vi "Turret_Execute.vi"() -> ()   [LabVIEW 2019]
uses:
  Turret_States.ctl
  Utility VIs/Basic_Motor_Modes.ctl
  Globals/Turret_Globals.vi
  Globals/Sensor_Values.vi
panel:
  in  "Disable Edge Safeties?":bool
  out "Waveform Chart":cluster{"Goal Wheel Position":dbl, dbl}(graph)
  in  "Kp_Degrees":dbl=0.07
  in  "Kd Aim":dbl=0.001
  in  "Ki Aim":dbl=1e-05
  out "Turret_Spin_Speed":dbl
  in  "Kp Aim":dbl=0.06
  # "e"
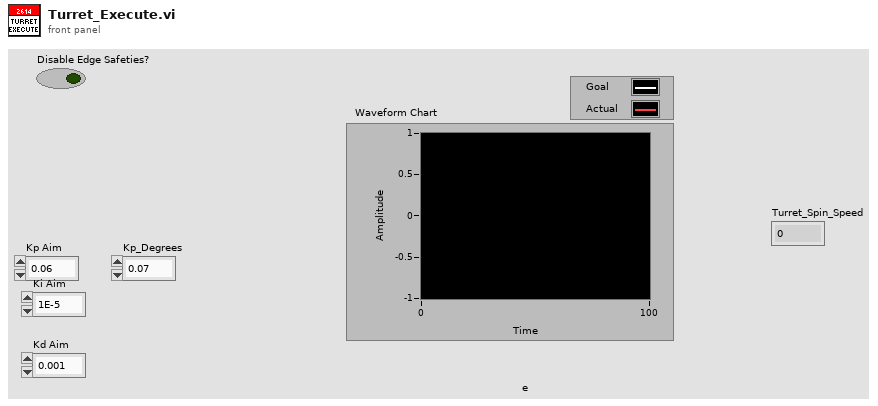
[diagram p1: front panel]
types:
  T1 = typedef "Turret_States.ctl" = enum16{"Manual_Percent_Voltage", "Manual_Speed_Control", "Auto-Target", "Command_TurnToPosition", "Command_Auto_Target", "GoToZero"}
  T2 = typedef "Basic_Motor_Modes.ctl" = enum16{"Percent_Voltage", "Speed_Control", "Position_Control", "Current"}
  T3 = typedef "Turret_Cluster.ctl" = cluster{"Auto-Target?":bool, "Control_State":T1, "Turret_Spin_Speed":dbl, "Turret_Spin_Speed_Control?":bool, "Step":dbl, "Auto_Notifier":refnum<notifier>, "GoToZero?":bool, "Parameters":dbl[]}
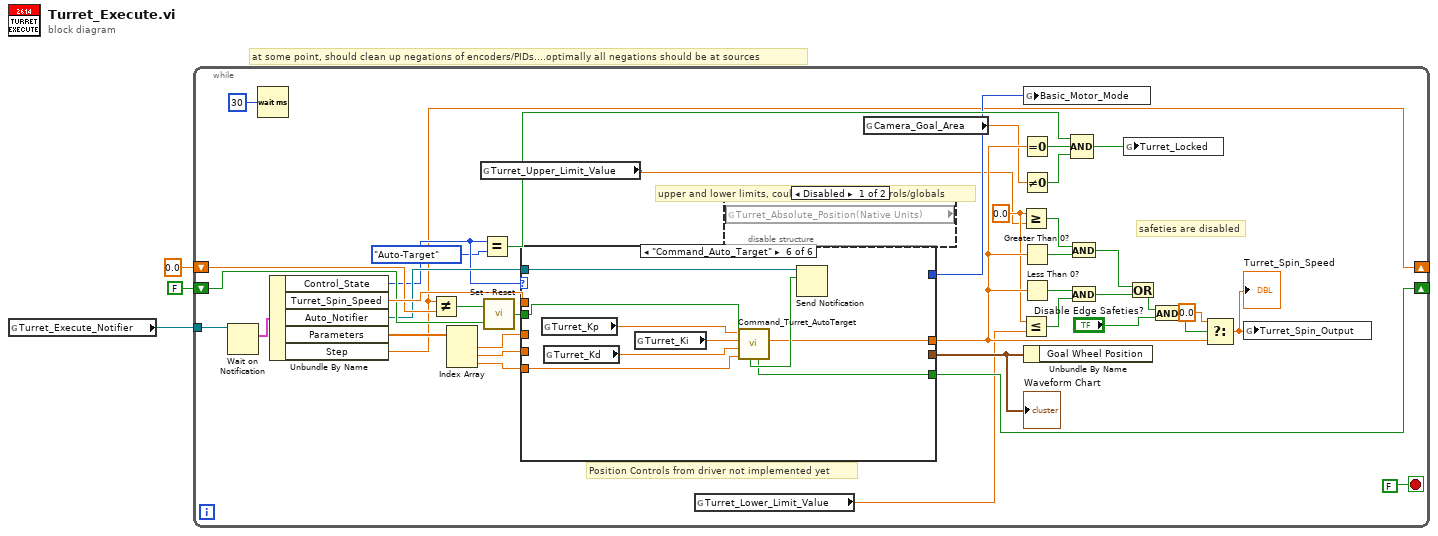
[diagram p0: block diagram]
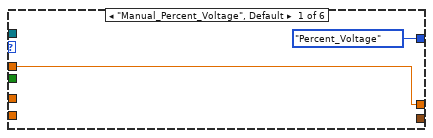
[diagram p3: hidden frame]
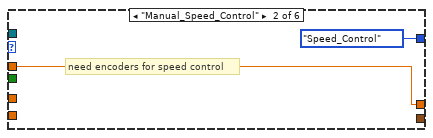
[diagram p4: hidden frame]
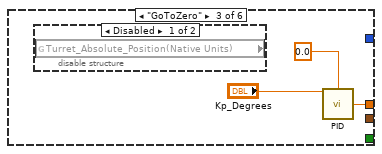
[diagram p5: hidden frame]
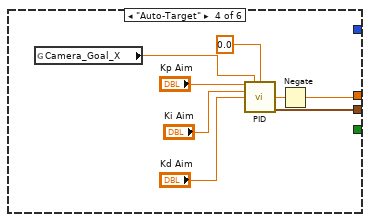
[diagram p7: hidden frame]
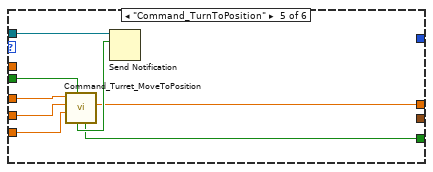
[diagram p8: hidden frame]
diagram:
  # "at some point, should clean up negations of encoders/PIDs....optimally all negations should be at sources"
  n1 = global read "Turret_Globals.vi" "Turret_Execute_Notifier"() -> (w3:refnum<notifier>)
  n2 = while {
    tunnel: w3 -> [w42]
    shift-right: [w6] -> _
    shift-left: 0.0 ("Step") -> [w31]
    shift-right: [w25] -> _
    shift-left: FALSE ("Output") -> [w29]
    stop <- FALSE stop-if-true
    w10 = 0.0 ("x")
    # "safeties are disabled"
    # "Position Controls from driver not implemented yet"
    # "upper and lower limits, could be made into controls/globals"
    n3 = Wait on Notification(notifier=w42) -> (notification=w41:T3)  [unwired: 3 in, 3 out]
    n4 = Wait (ms)(milliseconds to wait=u32 30) -> ()  [unwired: 1 out]
    n5 = Unbundle By Name(w41) -> ("Control_State"=w24:T1, "Turret_Spin_Speed"=w40:dbl, "Auto_Notifier"=w26:refnum<notifier>, "Parameters"=w28:dbl[], "Step"=w6:dbl)
    n6 = Not Equal?(x=w6, y=w31) -> (x != y?=w30:bool)
    n7 = Index Array(array=w28) -> (element #1=w9:dbl, element #2=w8:dbl, element #3=w7:dbl)  [unwired: 3 in]
    n8 = global read "Sensor_Values.vi" "Turret_Upper_Limit_Value"() -> (w5:dbl)
    n9 = Equal?(x=w24, y=Turret_States."Auto-Target") -> (x = y?=w20:bool)
    n10 = call "Set - Reset.vi"("Reset"=w29, "Set"=w30) -> ("Output"=w27:bool)
    n11 = case shown="\"Command_Auto_Target\"" w24 {
      tunnel: w40 -> [w45 w47 _ _ _ _]
      tunnel: [w45 w47 w48 w51 w59 w70] -> w22
      tunnel: w9 -> [_ _ _ _ w66 _]
      tunnel: w8 -> [_ _ _ _ w65 _]
      tunnel: w7 -> [_ _ _ _ w64 w75]
      tunnel: w27 -> [_ _ _ _ w63 w74]
      tunnel: w26 -> [_ _ _ _ w62 w73]
      tunnel: [_ _ _ _ w60 w71] -> w25
      tunnel: [_ _ _ w53 _ _] -> w16
      tunnel: [Basic_Motor_Modes."Percent_Voltage" ("Motor_Mode") Basic_Motor_Modes."Speed_Control" ("Motor_Mode") _ _ _ _] -> w14
      frame "Manual_Percent_Voltage", Default {
      }
      frame "Manual_Speed_Control" {
        # "need encoders for speed control"
      }
      frame "GoToZero" {
        n12 = disable-structure shown="Disabled" {
          frame Disabled {
            n13 = global read "Sensor_Values.vi" "Turret_Absolute_Position(Native Units)"() -> ()  [unwired: 1 out]
          }
          frame Enabled {
          }
        }
        n14 = call "PID.vi"("Kp"="Kp_Degrees", "Goal"=0.0) -> ("Command"=w48:dbl)  [unwired: 11 in, 2 out]
      }
      frame "Auto-Target" {
        n15 = global read "Sensor_Values.vi" "Camera_Goal_X"() -> (w56:dbl)
        n16 = call "PID.vi"("Kp"="Kp Aim", "Process Variable"=w56, "Goal"=0.0, "Ki"="Ki Aim", "Kd"="Kd Aim") -> ("Command"=w52:dbl, "PID Tracking"=w53:cluster{"Goal Wheel Position":dbl, dbl})  [unwired: 8 in, 1 out]
        n17 = Negate(x=w52) -> (-x=w51:dbl)
      }
      frame "Command_TurnToPosition" {
        n18 = call "Command_Turret_MoveToPosition.vi"("Startup"=w63, "Timeout"=w64, "Speed"=w65, "Goal_Position"=w66) -> ("Turret_Speed"=w59:dbl, "Reint"=w60:bool, "Completed"=w61:bool)  [unwired: 5 in]
        n19 = Send Notification(notification=w61, notifier=w62) -> ()  [unwired: 1 in, 2 out]
      }
      frame "Command_Auto_Target" {
        n20 = global read "Sensor_Values.vi" "Turret_Kp"() -> (w69:dbl)
        n21 = global read "Sensor_Values.vi" "Turret_Kd"() -> (w67:dbl)
        n22 = global read "Sensor_Values.vi" "Turret_Ki"() -> (w68:dbl)
        n23 = call "Command_Turret_AutoTarget.vi"("Startup"=w74, "Timeout"=w75, "Kd"=w67, "Ki"=w68, "Kp"=w69) -> ("Turret_Speed"=w70:dbl, "Reint"=w71:bool, "Completed"=w72:bool)  [unwired: 4 in]
        n24 = Send Notification(notification=w72, notifier=w73) -> ()  [unwired: 1 in, 2 out]
      }
    }
    "Waveform Chart" <- w16
    n25 = global read "Sensor_Values.vi" "Turret_Lower_Limit_Value"() -> (w4:dbl)
    n26 = disable-structure shown="Disabled" {
      frame Disabled {
        n27 = global read "Sensor_Values.vi" "Turret_Absolute_Position(Native Units)"() -> ()  [unwired: 1 out]
      }
      frame Enabled {
      }
    }
    n28 = global read "Sensor_Values.vi" "Camera_Goal_Area"() -> (w18:dbl)
    n29 = Greater Or Equal?(x=w10, y=w5) -> (x >= y?=w39:bool)
    n30 = Less Or Equal?(x=w10, y=w4) -> (x <= y?=w32:bool)
    n31 = Equal To 0?(x=w22) -> (x = 0?=w19:bool)
    n32 = Not Equal To 0?(x=w18) -> (x != 0?=w17:bool)
    n33 = Greater Than 0?(x=w22) -> (x > 0?=w38:bool)
    n34 = Less Than 0?(x=w22) -> (x < 0?=w37:bool)
    n35 = global write "Turret_Globals.vi" "Basic_Motor_Mode"(w14) -> ()
    n36 = Unbundle By Name(w16) -> ()  [unwired: 1 out]
    n37 = And(x=w39, y=w38) -> (x .and. y?=w35:bool)
    n38 = And(x=w37, y=w32) -> (x .and. y?=w36:bool)
    n39 = Compound Arithmetic op=AND(w20, w19, w17) -> (w21:bool)
    n40 = global write "Turret_Globals.vi" "Turret_Locked"(w21) -> ()
    n41 = Or(x=w35, y=w36) -> (x .or. y?=w13:bool)
    n42 = And(x=w13, y="Disable Edge Safeties?") -> (x .and. y?=w11:bool)
    n43 = Select(t=0.0, s=w11, f=w22) -> (s? t:f=w15:dbl)
    "Turret_Spin_Speed" <- w15
    n44 = global write "Turret_Globals.vi" "Turret_Spin_Output"(w15) -> ()
  }
